vi "AutoDetector_GetPeak.vi"(6 "AutoDV Info":T1, 8 "error in":errorcluster, 9 "CalOption":enum32{"Positive", "Negative"}(radio), 10 "Model Name":T3=enum."IONICS 3Q 210", 11 "Current Results":string[][](table) caption="08/02/2016 14:17:04") -> (0 "error in":errorcluster, 3 "AutoDV Info Out":T1)   [LabVIEW 2015]
uses:
  Type/_Instrument Model.ctl
  Controls/Auto-Detector Bias Info.ctl
  Controls/Auto-Detector Peak Info.ctl
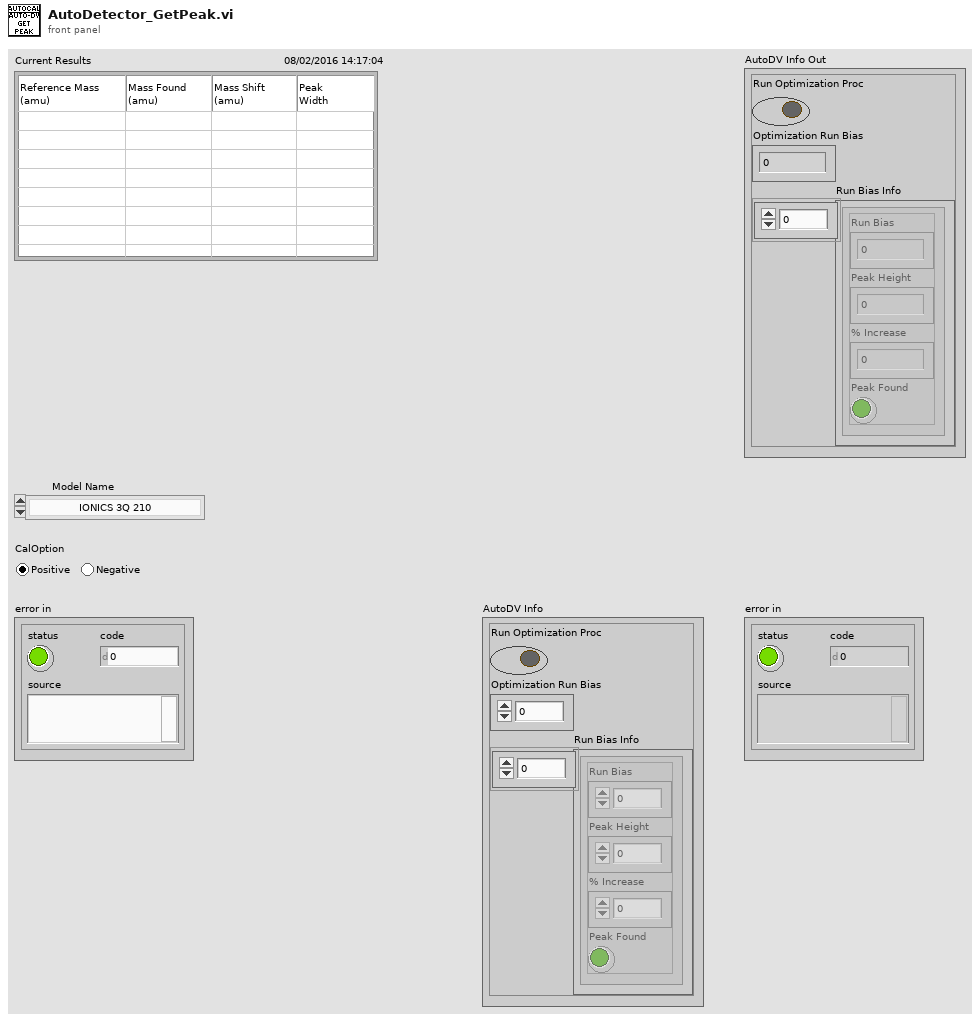
[diagram p1: front panel]
types:
  T1 = typedef "Auto-Detector Bias Info.ctl" = cluster{"Run Optimization Proc":bool, "Optimization Run Bias":u32, "Run Bias Info":T2[]}
  T2 = typedef "Auto-Detector Peak Info.ctl" = cluster{"Run Bias":u32, "Peak Height":dbl, "% Increase":dbl, "Peak Found":bool}
  T3 = typedef "_Instrument Model.ctl" = enum16{"QSight 110", "QSight 120", "QSight 210", "QSight 220", "IONICS 3Q 110", "IONICS 3Q 120", "IONICS 3Q 210", "IONICS 3Q 220", "IONICS 3Q 310", "IONICS 3Q 320", "Simulation (Single Source)", "Simulation (Dual Source)"}
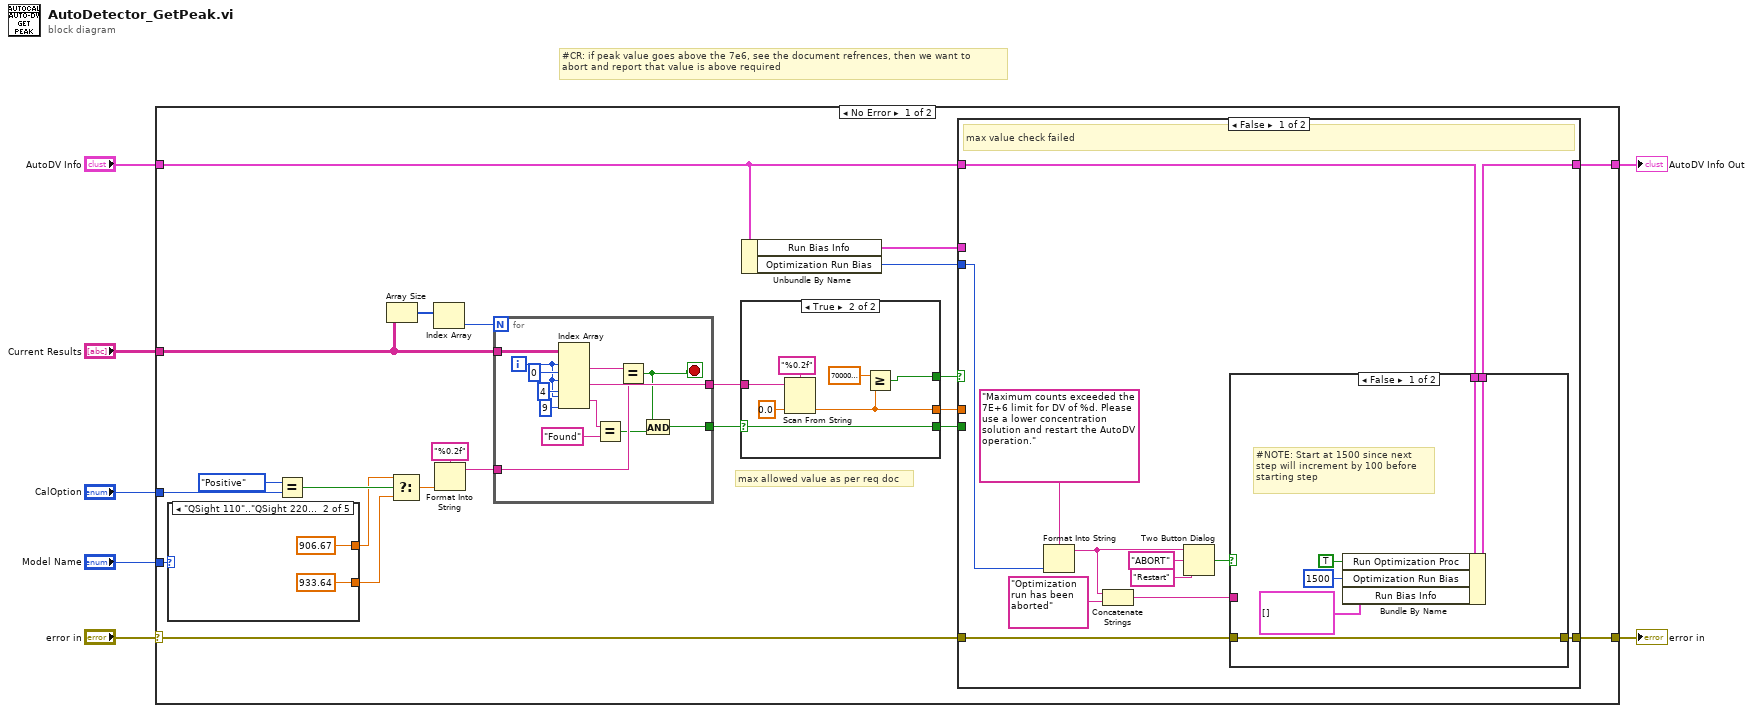
[diagram p0: block diagram]
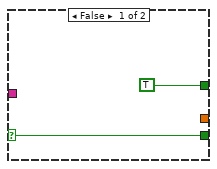
[diagram p2: hidden frame]
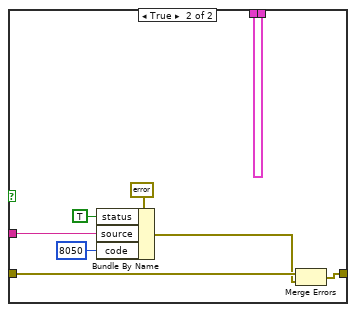
[diagram p3: hidden frame]
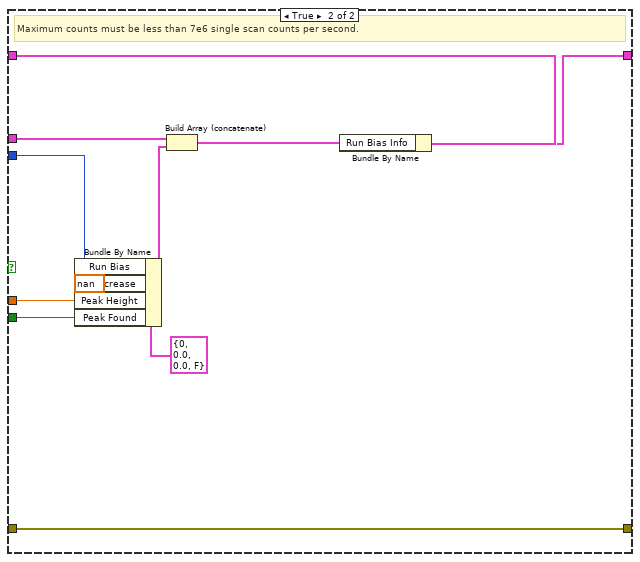
[diagram p4: hidden frame]
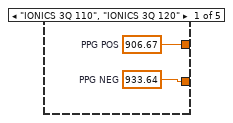
[diagram p5: hidden frame]
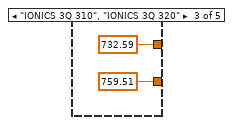
[diagram p6: hidden frame]
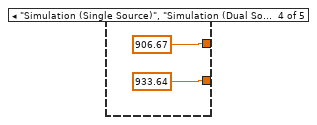
[diagram p7: hidden frame]
diagram:
  # "#CR: if peak value goes above the 7e6, see the document refrences, then we want to \nabort and report that value is above required"
  n1 = case shown="No Error" "error in" {
    selector: "error in" -> [w14 w99]
    tunnel: "Model Name" -> [w30 _]
    tunnel: "Current Results" -> [w29 _]
    tunnel: "CalOption" -> [w26 _]
    tunnel: [w15 w99] -> w4
    tunnel: "AutoDV Info" -> [w12 w98]
    tunnel: [w11 w98] -> w1
    frame No Error {
      # "max allowed value as per req doc"
      n2 = case shown="\"QSight 110\"..\"QSight 220\", \"IONICS 3Q 210\", \"IONICS 3Q 220\"" w30 {
        tunnel: [w91 906.67 ("PPG POS") 732.59 ("PPG POS") 906.67 ("PPG POS") _] -> w23
        tunnel: [w90 933.64 ("PPG NEG") 759.51 ("PPG NEG") 933.64 ("PPG NEG") _] -> w22
        frame "IONICS 3Q 110", "IONICS 3Q 120" {
          w90 = 933.64  # PPG NEG
          w91 = 906.67  # PPG POS
        }
        frame "QSight 110".."QSight 220", "IONICS 3Q 210", "IONICS 3Q 220" {
        }
        frame "IONICS 3Q 310", "IONICS 3Q 320" {
        }
        frame "Simulation (Single Source)", "Simulation (Dual Source)" {
        }
        frame Default {
        }
      }
      n3 = Equal?(x=enum32{"Positive", "Negative"}."Positive", y=w26) -> (x = y?=w24:bool)
      n4 = Array Size(array=w29) -> (size(s)=w28:i32[])
      n5 = Select(t=w23, s=w24, f=w22) -> (s? t:f=w21:dbl)
      n6 = Index Array(array=w28) -> (element=w27:i32)  [unwired: 1 in]
      n7 = Format Into String(format string="%0.2f", w21) -> (resulting string=w19:string)  [unwired: 2 in, 1 out]
      n8 = for {
        N: w27 -> [_]
        tunnel: w29 -> [w89]
        tunnel: [w86] -> w18
        tunnel: w19 -> [w80]
        tunnel: [w77] -> w10
        i -> [w84]
        stop <- w79 stop-if-true
        n9 = Index Array(array=w89, index (row) #1=w84, index (col) #1=0 ("disabled index (col)"), index (row) #2=w84, index (col) #2=4 ("disabled index (col)"), index (row) #3=w84, index (col) #3=9 ("index (col)")) -> (element #1=w82:string, element #2=w86:string, element #3=w81:string)
        n10 = Equal?(x=w81, y="Found") -> (x = y?=w78:bool)
        n11 = Equal?(x=w82, y=w80) -> (x = y?=w79:bool)
        n12 = And(x=w79, y=w78) -> (x .and. y?=w77:bool)
      }
      n13 = case shown="True" w10 {
        selector: w10 -> [w32 w34]
        tunnel: w18 -> [_ w37]
        tunnel: [_ w36] -> w13
        tunnel: [w32 w34] -> w9
        tunnel: [TRUE w33] -> w8
        frame False {
        }
        frame True {
          n14 = Scan From String(format string="%0.2f", input string=w37, default 1=0.0 ("default value 1")) -> (output 1=w36:dbl)  [unwired: 2 in, 3 out]
          n15 = Greater Or Equal?(x=70000000.0, y=w36) -> (x >= y?=w33:bool)
        }
      }
      n16 = Unbundle By Name(w12) -> ("Run Bias Info"=w17:T2[], "Optimization Run Bias"=w16:u32)
      n17 = case shown="False" w8 {
        tunnel: w9 -> [_ w76]
        tunnel: w13 -> [_ w75]
        tunnel: w17 -> [_ w74]
        tunnel: w16 -> [w50 w69]
        tunnel: [w48 w68] -> w15
        tunnel: w14 -> [w49 w68]
        tunnel: w12 -> [w41 w67]
        tunnel: [w40 w66] -> w11
        frame False {
          # "max value check failed"
          n18 = Format Into String(format string="Maximum counts exceeded the 7E+6 limit for DV of %d. Please use a lower concentration solution and restart the AutoDV operation." ("source"), w50) -> (resulting string=w44:string)  [unwired: 2 in, 1 out]
          n19 = Concatenate Strings(w44, "Optimization run has been aborted" ("string")) -> (w43:string)
          n20 = Two Button Dialog(message=w44, 1:"Restart" ("F button name (\"Cancel\")"), 2:"ABORT" ("T button name (\"OK\")")) -> (T button?=w42:bool)
          n21 = case shown="False" w42 {
            tunnel: w49 -> [w57 w63]
            tunnel: [w57 w62] -> w48
            tunnel: w43 -> [_ w60]
            tunnel: w41 -> [w56 w58]
            tunnel: [w55 w58] -> w40
            frame False {
              # "#NOTE: Start at 1500 since next \nstep will increment by 100 before \nstarting step"
              n22 = Bundle By Name(cluster=w56, "Run Optimization Proc"=TRUE, "Optimization Run Bias"=u32 1500, "Run Bias Info"=T2[] []) -> (w55:T1)
            }
            frame True {
              n23 = Bundle By Name(cluster=errorcluster {"status"=FALSE, "code"=0, "source"=""} ("error IO"), "status"=TRUE, "source"=w60, "code"=8050) -> (w61:errorcluster)
              n24 = Merge Errors(w63, w61) -> (w62:errorcluster)
            }
          }
        }
        frame True {
          # "Maximum counts must be less than 7e6 single scan counts per second."
          n25 = Bundle By Name(cluster=T2 {"Run Bias"=0, "Peak Height"=0.0, "% Increase"=0.0, "Peak Found"=FALSE} ("Run Bias"), "Run Bias"=w69, "% Increase"=nan, "Peak Height"=w75, "Peak Found"=w76) -> (w71:T2)
          n26 = Build Array (concatenate)(w74, w71) -> (w73:T2[])
          n27 = Bundle By Name(cluster=w67, "Run Bias Info"=w73) -> (w66:T1)
        }
      }
    }
    frame Error {
    }
  }
  "error in" <- w4
  "AutoDV Info Out" <- w1
